vi "filtra.vi"(1 "Numeric":i32, 2 "Data 2":waveform(dbl)) -> (0 "Data":waveform(dbl))   [LabVIEW 2010]
uses:
  <vilib>/Analysis/3filter.llb/Equi-Ripple BandPass (DBL).vi
  <vilib>/Analysis/NI_AALBase.lvlib
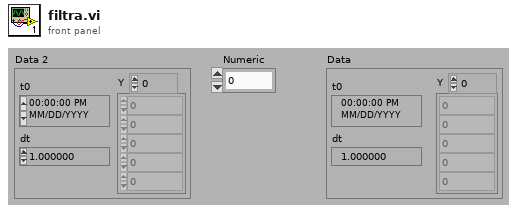
[diagram p1: front panel]
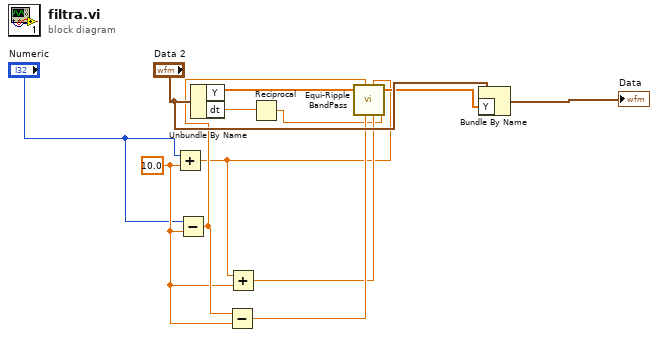
[diagram p0: block diagram]
diagram:
  w5 = 10.0 ("y")
  n1 = Add(x="Numeric", y=w5) -> (x+y=w6:dbl)
  n2 = Subtract(x="Numeric", y=w5) -> (x-y=w7:dbl)
  n3 = Unbundle By Name("Data 2") -> ("Y"=w2:dbl[], "dt"=w1:dbl)
  n4 = Subtract(x=w7, y=w5) -> (x-y=w9:dbl)
  n5 = Add(x=w6, y=w5) -> (x+y=w8:dbl)
  n6 = Reciprocal(x=w1) -> (1/x=w3:dbl)
  n7 = call-poly <vilib>:"Equi-Ripple BandPass.vi"("X"=w2, "lower pass freq"=w7, "lower stop freq"=w9, "higher pass freq"=w6, "higher stop freq"=w8, "sampling freq: fs"=w3) -> ("Filtered X"=w10:dbl[])  [unwired: 2 in, 1 out]
  n8 = Bundle By Name(cluster="Data 2", "Y"=w10) -> (→"Data":waveform(dbl))
